vi "CSConnect.SetOnOff.vi"(0 "i ref in":refnum<vi>, 2 "In-channel number":i32, 3 "On?":bool=TRUE, 5 "error in (no error)":errorcluster) -> (14 "i ref out":refnum<vi>, 19 "error out":errorcluster)   [LabVIEW 2014, in "CSConnect.lvlib"]
doc: "Switches all Out-channels belonging to an In-Channel On or Off.\n\nLicense Agreement for this software:\n\nCopyright (C)\nGesellschaft für Schwerionenforschung, GSI\nPlanckstr. 1\n64291 Darmstadt\nGermany\n\nContact: D.Beck@gsi.de \n\nThis program is free software; you can redistribute it and/or modify it under the terms of the \nGNU General Public License as published by the Free Software Foundation; either version 2 of \nthe license, or (at your option) any later version.\n\nThis program is distributed in the hope that it will be useful, but WITHOUT ANY WARRANTY; \nwithout even the implied warranty of MERCHANTABILITY or FITNESS FOR A PARTICULAR PURPOSE. See the GNU General License for more details (http://www.gnu.org).\n\nGesellschaft für Schwerionenforschung, GSI\nPlanckstr. 1, 64291 Darmstadt, Germany\nFor all questions and ideas contact: M.Richter@gsi.de, H.Brand@gsi.de or D.Beck@gsi.de.\nLast update: 16-JUN-2004"
uses:
  CSConnect.lvlib
  CS_Core/CSSystem/CoreLib/CoreLib.int 2 byte array.vi
  CS_Core/CSSystem/CoreLib/CoreLib.short 2 byte array.vi
  CS_Core/BaseProcess/BaseProcess.lvlib
  CS_Core/CSSystem/CoreLib/CoreLib.lvlib
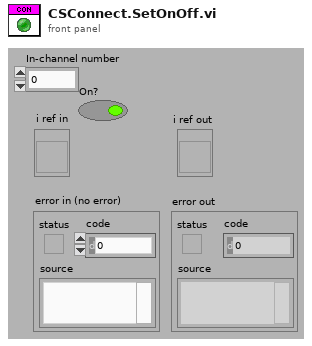
[diagram p1: front panel]
types:
  T1 = typedef "CSConnect.lvlib/CSConnect.i attribute.ctl" = cluster{"In-Array":cluster{"Alias":string, "Value":dbl, "neededOuts":bool[]}[], "Out-Array":cluster{"ObjectName":string, "VoltFunctionName":string, "OnOffFunctionName":string, "Channel":string, "Calculation-Formula":string}[], "OutChannelsID":i32, "InOutMatrixID":i32}
  T2 = cluster{"Alias":string, "Value":dbl, "neededOuts":bool[]}[]
  T3 = cluster{"ObjectName":string, "VoltFunctionName":string, "OnOffFunctionName":string, "Channel":string, "Calculation-Formula":string}[]
  T4 = cluster{"Alias":string, "Value":dbl, "neededOuts":bool[]}
  T5 = typedef "CoreDefs.rawDataType.ctl" = i8[]
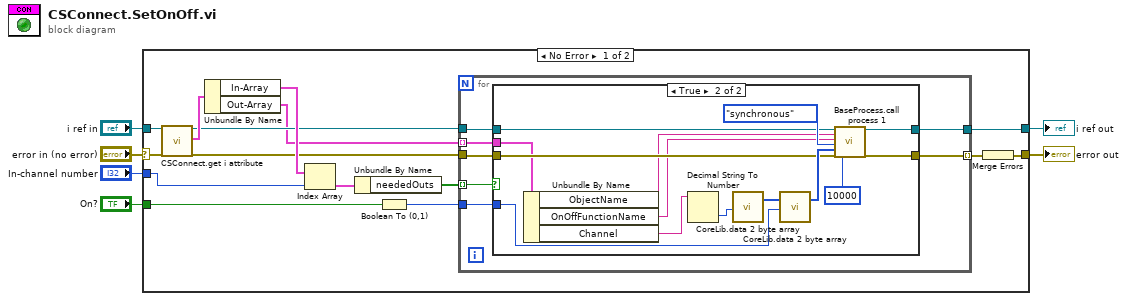
[diagram p0: block diagram]
diagram:
  n1 = case shown="No Error" "error in (no error)" {
    selector: "error in (no error)" -> [w20 w45]
    tunnel: [w7 w45] -> w6
    tunnel: [w8 w46] -> w4
    tunnel: "i ref in" -> [w21 w46]
    tunnel: "In-channel number" -> [w18 _]
    tunnel: "On?" -> [w11 _]
    frame No Error {
      n2 = call "CSConnect.get i attribute.vi"("i ref in"=w21, "error in (no error)"=w20) -> ("i ref out"=w13:refnum<vi>, "i attribute"=w19:T1, "error out"=w14:errorcluster)  [unwired: 15 in]
      n3 = Unbundle By Name(w19) -> ("In-Array"=w17:T2, "Out-Array"=w12:T3)
      n4 = Index Array(array=w17, index=w18) -> (element=w16:T4)
      n5 = Unbundle By Name(w16) -> ("neededOuts"=w15:bool[])
      n6 = Boolean To (0,1)(Boolean=w11) -> (0, 1=w10:i16)
      n7 = for {
        tunnel: w15 -> [w26] mode=indexing
        tunnel: w10 -> [w25]
        tunnel: w14 -> [w28]
        tunnel: w13 -> [w27]
        tunnel: w12 -> [w24] mode=indexing
        tunnel: [w23] -> w9 mode=indexing
        tunnel: [w22] -> w8
        n8 = case shown="True" w26 {
          tunnel: w28 -> [w29 w39]
          tunnel: w27 -> [w30 w38]
          tunnel: w25 -> [_ w33]
          tunnel: w24 -> [_ w37]
          tunnel: [w29 w32] -> w23
          tunnel: [w30 w31] -> w22
          frame False {
          }
          frame True {
            n9 = Unbundle By Name(w37) -> ("ObjectName"=w36:string, "OnOffFunctionName"=w35:string, "Channel"=w34:string)
            n10 = Decimal String To Number(string=w34) -> (number=w40:i32)  [unwired: 2 in, 1 out]
            n11 = call-poly "CoreLib.data 2 byte array.vi"("i32"=w40) -> ("byteArray out"=w43:T5)  [unwired: 18 in]
            n12 = call-poly "CoreLib.data 2 byte array.vi"("byteArray"=w43, "i16"=w33) -> ("byteArray out"=w42:T5)  [unwired: 17 in]
            n13 = call "BaseProcess.call process 1.vi"("i ref in"=w38, "Object"=w36, "Selector"=w35, "CallType"=enum16{"simple", "synchronous", "asynchronous"}."synchronous", "Data"=w42, "error in (no error)"=w39, "timeout (ms)"=10000) -> ("i ref out"=w31:refnum<vi>, "error out"=w32:errorcluster)  [unwired: 10 in, 1 out]
          }
        }
      }
      n14 = Merge Errors(w9) -> (w7:errorcluster)
    }
    frame Error {
    }
  }
  "error out" <- w6
  "i ref out" <- w4
